vi "Eichung_R5.vi"(11 "R (Ohm)":dbl=4203.0 format="%.5f") -> (3 "T (K)":dbl=0.29275308045912907 format="%.6f")   [LabVIEW 2019]
panel:
  in  "T (K) 2":dbl=0.1 format="%.5f"
  out "R (Ohm) 2":dbl=inf format="%.6f"
  in  "log poly fit coeffiecients R(T)":T1={"0"=1.0, "1"=1.0, "2"=1.0, "3"=1.0, "4"=1.0, "5"=1.0, "6"=1.0, "7"=1.0, "8"=1.0, "9"=1.0} {"9" format="%.16f"; "8" format="%.16f"; "7" format="%.16f"; "6" format="%.16f"; "5" format="%.14f"; "4" format="%.14f"; "3" format="%.14f"; "2" format="%.13f"; "1" format="%.13f"; "0" format="%.13f"}
  in  "cluster":T1={"0"=92.48879464, "1"=-130.710141, "2"=77.11444301, "3"=-24.20318633, "4"=4.003562644, "5"=-0.1351479966, "6"=-0.1080121635, "7"=0.03098235003, "8"=-0.004003115845, "9"=0.0002089085669} {"0" format="%#_14g"; "1" format="%#_14g"; "2" format="%#_14g"; "3" format="%#_14g"; "4" format="%#_14g"; "5" format="%#_14g"; "6" format="%#_14g"; "7" format="%#_14g"; "8" format="%#_14g"; "9" format="%#_14g"}
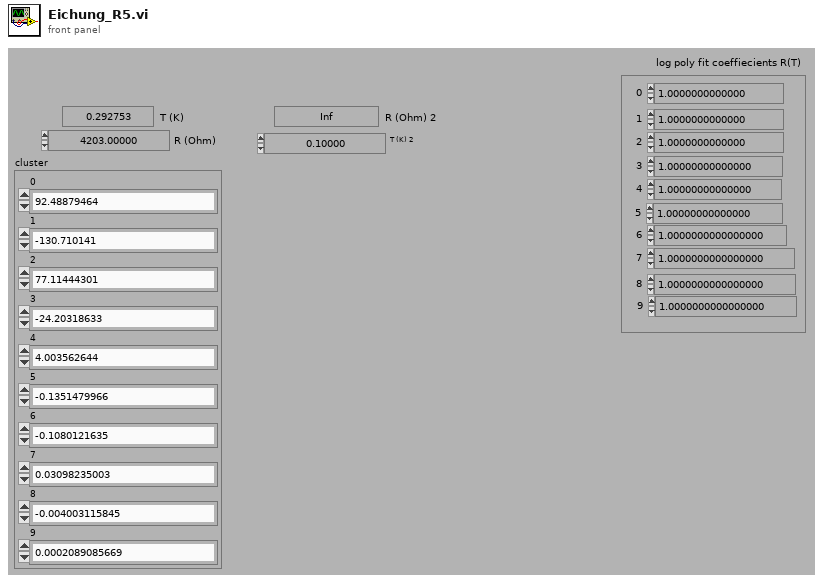
[diagram p1: front panel]
types:
  T1 = cluster{"0":dbl, "1":dbl, "2":dbl, "3":dbl, "4":dbl, "5":dbl, "6":dbl, "7":dbl, "8":dbl, "9":dbl}
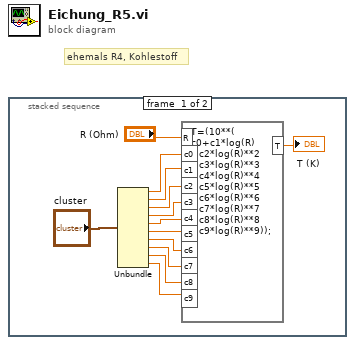
[diagram p0: block diagram]
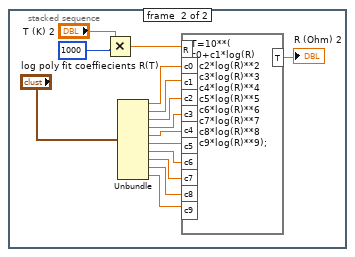
[diagram p2: hidden frame]
diagram:
  # "ehemals R4, Kohlestoff"
  n1 = stacked-sequence {
    frame #0 {
      n2 = Unbundle("cluster") -> ("0"=w2:dbl, "1"=w3:dbl, "2"=w4:dbl, "3"=w5:dbl, "4"=w6:dbl, "5"=w7:dbl, "6"=w8:dbl, "7"=w9:dbl, "8"=w10:dbl, "9"=w11:dbl)
      n3 = formula code="T=(10**(\nc0+c1*log(R)\n+c2*log(R)**2\n+c3*log(R)**3\n+c4*log(R)**4\n+c5*log(R)**5\n+c6*log(R)**6\n+c7*log(R)**7\n+c8*log(R)**8\n+c9*log(R)**9));"("R"="R (Ohm)", "c0"=w2, "c1"=w3, "c2"=w4, "c3"=w5, "c4"=w6, "c5"=w7, "c6"=w8, "c7"=w9, "c8"=w10, "c9"=w11) -> ("T"=→"T (K)":dbl)
    }
    frame #1 {
      n4 = Multiply(x="T (K) 2", y=1000) -> (x*y=w15:dbl)
      n5 = Unbundle("log poly fit coeffiecients R(T)") -> ("0"=w19:dbl, "1"=w20:dbl, "2"=w21:dbl, "3"=w22:dbl, "4"=w23:dbl, "5"=w24:dbl, "6"=w25:dbl, "7"=w26:dbl, "8"=w27:dbl, "9"=w28:dbl)
      n6 = formula code="T=10**(\nc0+c1*log(R)\n+c2*log(R)**2\n+c3*log(R)**3\n+c4*log(R)**4\n+c5*log(R)**5\n+c6*log(R)**6\n+c7*log(R)**7\n+c8*log(R)**8\n+c9*log(R)**9);"("R"=w15, "c0"=w19, "c1"=w20, "c2"=w21, "c3"=w22, "c4"=w23, "c5"=w24, "c6"=w25, "c7"=w26, "c8"=w27, "c9"=w28) -> ("T"=→"R (Ohm) 2":dbl)
    }
  }
